vi "crio_vi.vi"() -> ()   [LabVIEW 2014]
uses:
  <vilib>/Platform/TimedLoop/XDataNode/timing_clust.ctl
  <vilib>/Platform/TimedLoop/XDataNode/nitl_modes.ctl
  <vilib>/Platform/TimedLoop/XDataNode/wakeup.ctl
  <vilib>/imath/engines/lvmath2/RunTimeEngine/NodeEndStatement/NIMS_NodeEndStatement_Output.vi
  <instcachedir>/0/NIMS_NodeEndStatement_Output_53EC0D466D134D7ABD903AC30B43404B.lvgen/NIMS_NodeEndStatement_Output_53EC0D466D134D7ABD903AC30B43404B_001.vi
  <vilib>/imath/engines/lvmath2/RunTimeEngine/ErrorHandling/NIMS_Finalize Error.vi
  <vilib>/platform/TimedLoop/XDataNode/XDataNode.xnode
  <vilib>/Platform/TimedLoop/XDataNode/XDNodeRunTimeDep.lvlib
panel:
  out "Waveform Chart":dbl(graph)
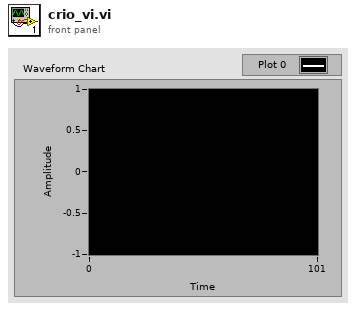
[diagram p1: front panel]
types:
  T1 = typedef "XDNodeRunTimeDep.lvlib/timing_clust.ctl" = cluster{"Expected End [f-1]":u64, "Actual End [f-1]":u64, "Finished Late? [f-1]":bool, "Expected End [i-1]":u64, "Actual End [i-1]":u64, "Finished Late? [i-1]":bool, "Expected Start [i]":u64, "Actual Start [i]":u64, "Expected Start [f]":u64, "Actual Start [f]":u64, "Source Name":string, "Structure Name":string, "Period":i64, "Deadline":i64, "Offset":i64, "Start":i64, "Priority":i32, "Timeout":i32, "Mode":T2, "Wakeup Reason":T3, "Error":errorcluster, "Source Type":string, "Secondary Source Type":string, "Global End Time":u64, "Global Start Time":u64, "Frame Duration":u64, "Iteration Duration":u64, "Assigned CPU":i32, "I/O Scan Engine Mode":u32}
  T2 = typedef "XDNodeRunTimeDep.lvlib/nitl_modes.ctl" = enum32{"No Change", "Process missed periods, maintain original phase", "Discard missed periods, maintain original phase", "Process missed periods, ignore original phase", "Discard missed periods, ignore original phase"}
  T3 = typedef "XDNodeRunTimeDep.lvlib/wakeup.ctl" = enum32{"Normal", "Aborted", "Asynchronous wakeup", "Timing source error", "Timed loop error", "Timeout"}
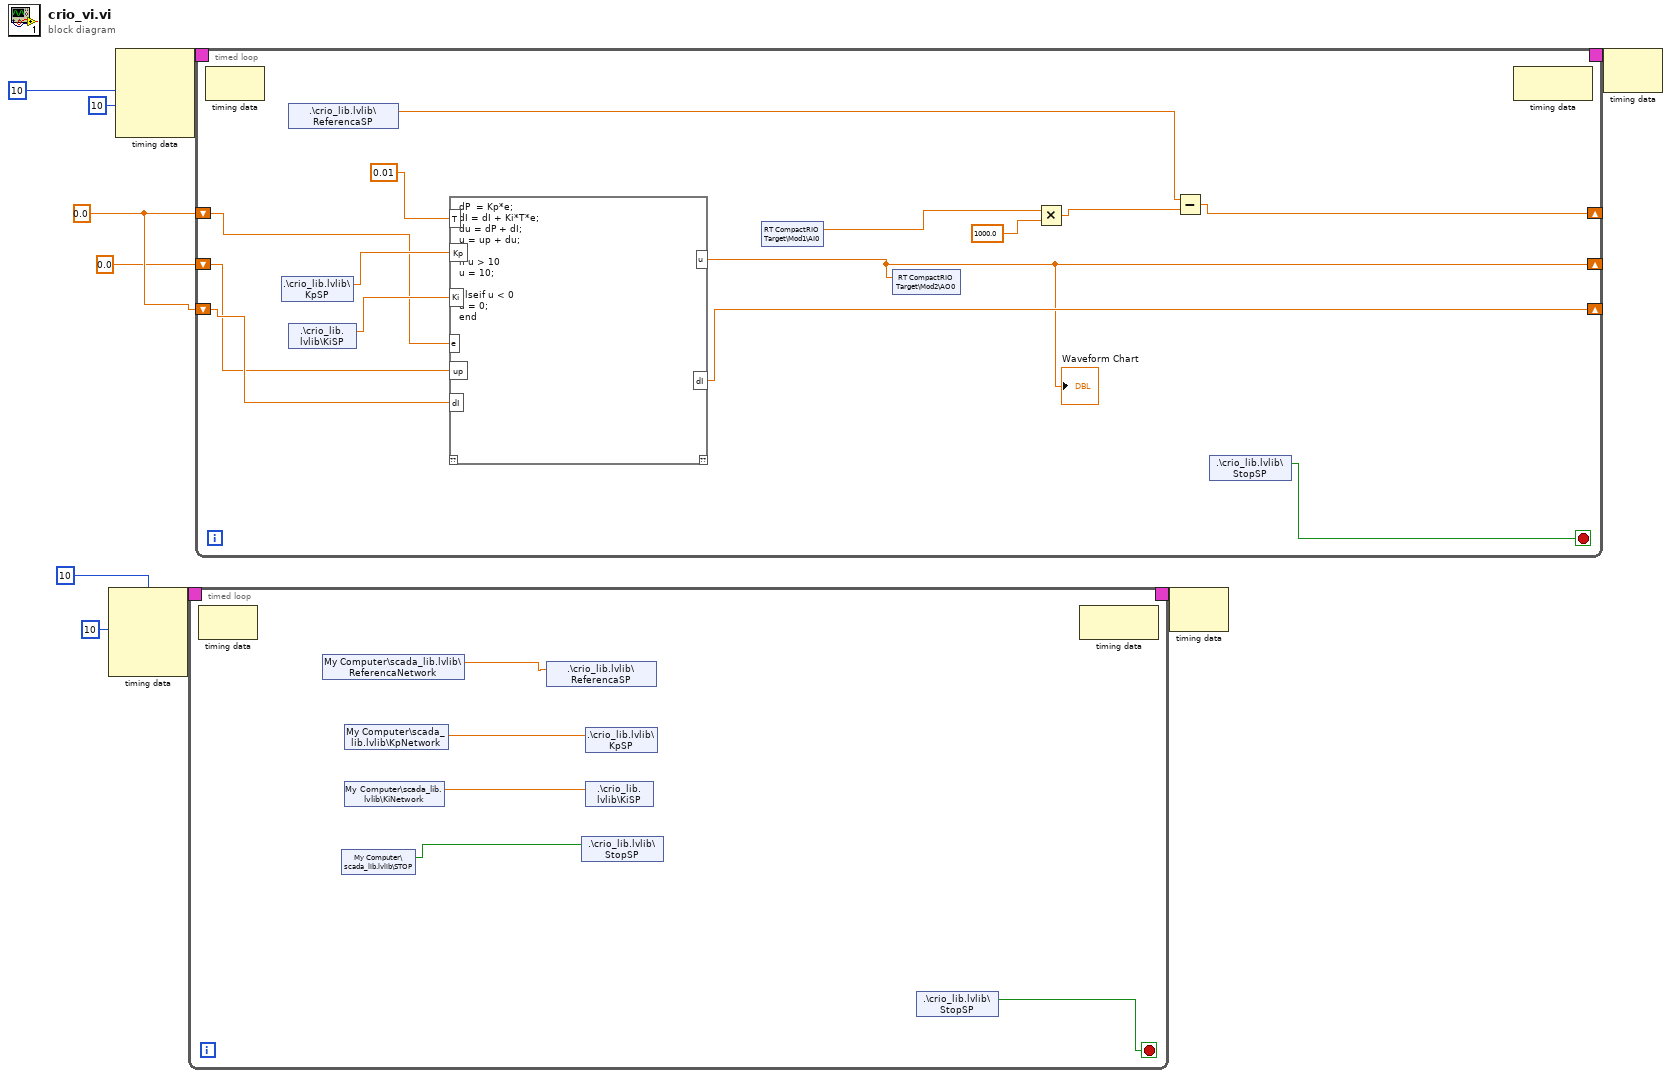
[diagram p0: block diagram]
diagram:
  w5 = 0.0
  n1 = node-c288(i64 10 ("Period"), 10 ("Priority")) -> (w7:T1)  [unwired: 2 in]
  n2 = node-c288(i64 10 ("Period"), 10 ("Priority")) -> (w10:T1)  [unwired: 2 in]
  n3 = timed-loop {
    timing: w7 -> [_]
    timing-out: [_] -> w6
    stop <- w12 stop-if-true
    n4 = node-c288() -> ()  [unwired: 1 in, 1 out]
    n5 = shared-variable "My Computer\\scada_lib.lvlib\\ReferencaNetwork"() -> (w11:dbl)  [unwired: 1 in, 1 out]
    n6 = shared-variable "My Computer\\scada_lib.lvlib\\STOP"() -> (w13:bool)  [unwired: 1 in, 1 out]
    n7 = shared-variable "My Computer\\scada_lib.lvlib\\KpNetwork"() -> (w14:dbl)  [unwired: 1 in, 1 out]
    n8 = shared-variable "My Computer\\scada_lib.lvlib\\KiNetwork"() -> (w15:dbl)  [unwired: 1 in, 1 out]
    n9 = shared-variable ".\\crio_lib.lvlib\\ReferencaSP"(w11) -> ()  [unwired: 1 in, 1 out]
    n10 = shared-variable ".\\crio_lib.lvlib\\StopSP"(w13) -> ()  [unwired: 1 in, 1 out]
    n11 = shared-variable ".\\crio_lib.lvlib\\KpSP"(w14) -> ()  [unwired: 1 in, 1 out]
    n12 = shared-variable ".\\crio_lib.lvlib\\KiSP"(w15) -> ()  [unwired: 1 in, 1 out]
    n13 = shared-variable ".\\crio_lib.lvlib\\StopSP"() -> (w12:bool)  [unwired: 1 in, 1 out]
    n14 = node-c288() -> ()  [unwired: 1 in, 1 out]
  }
  n15 = timed-loop {
    timing: w10 -> [_]
    timing-out: [_] -> w9
    shift-right: [w31] -> _
    shift-left: w5 -> [w26]
    shift-right: [w24] -> _
    shift-left: w5 -> [w25]
    shift-right: [w22] -> _
    shift-left: 0.0 ("u") -> [w23]
    stop <- w30 stop-if-true
    n16 = node-c288() -> ()  [unwired: 1 in, 1 out]
    n17 = shared-variable ".\\crio_lib.lvlib\\KpSP"() -> (w28:dbl)  [unwired: 1 in, 1 out]
    n18 = shared-variable ".\\crio_lib.lvlib\\ReferencaSP"() -> (w21:dbl)  [unwired: 1 in, 1 out]
    n19 = shared-variable ".\\crio_lib.lvlib\\KiSP"() -> (w27:dbl)  [unwired: 1 in, 1 out]
    n20 = mathscript code="dP  = Kp*e;\ndI = dI + Ki*T*e;\ndu = dP + dI;\nu = up + du;\n\nif u > 10\nu = 10;\n\nelseif u < 0\nu = 0;\nend"("T"=0.01 ("input variable"), "Kp"=w28, "Ki"=w27, "up"=w23, "e"=w26, "dI"=w25) -> ("dI"=w24:dbl, "u"=w22:dbl)  [unwired: 1 in, 1 out]
    "Waveform Chart" <- w22
    n21 = shared-variable "RT CompactRIO Target\\Mod1\\AI0"() -> (w20:dbl)  [unwired: 1 in, 1 out]
    n22 = shared-variable "RT CompactRIO Target\\Mod2\\AO0"(w22) -> ()  [unwired: 1 in, 1 out]
    n23 = Multiply(x=w20, y=1000.0) -> (x*y=w19:dbl)
    n24 = Subtract(x=w21, y=w19) -> (x-y=w31:dbl)
    n25 = shared-variable ".\\crio_lib.lvlib\\StopSP"() -> (w30:bool)  [unwired: 1 in, 1 out]
    n26 = node-c288() -> ()  [unwired: 1 in, 1 out]
  }
  n27 = node-c288(w6) -> ()  [unwired: 1 out]
  n28 = node-c288(w9) -> ()  [unwired: 1 out]
